vi "Player Info.vi"(11 "Tim_The_Enchanter in":refnum<class "Tim_The_Enchanter.lvclass">) -> (0 "Defeat Speech":string, 1 "Victory Speech":string, 2 "Name":string, 3 "Tim_The_Enchanter out":refnum<class "Tim_The_Enchanter.lvclass">)   [LabVIEW 2016, in "Tim_The_Enchanter.lvclass"]
uses:
  Tim_The_Enchanter.lvclass
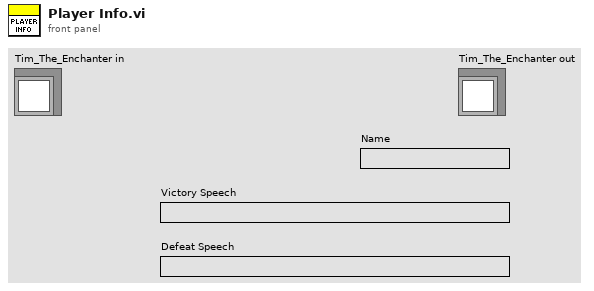
[diagram p1: front panel]
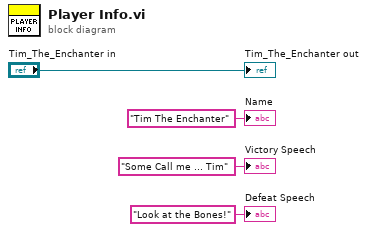
[diagram p0: block diagram]
diagram:
  "Tim_The_Enchanter out" <- "Tim_The_Enchanter in"
  "Name" <- "Tim The Enchanter" ("Name")
  "Victory Speech" <- "Some Call me ... Tim" ("Victory Speech")
  "Defeat Speech" <- "Look at the Bones!" ("Defeat Speech")
